vi "UDP Data Link RT Driver VI.vi"(7 "Operation":T1, 11 "Device Reference in":T2 format="%.0x") -> (0 "Error Code":i32)   [LabVIEW 2015, in "UDP Data Link Engine.lvlib"]
uses:
  UDP Data Link Engine.lvlib
  <vilib>/NI Veristand/Custom Device API/Custom Device Item Ref.ctl
  <vilib>/NI Veristand/Custom Device API/Hardware Interface Driver VI Operation.ctl
  <vilib>/NI Veristand/Custom Device API/Block Data Reference.ctl
  <vilib>/NI Veristand/Custom Device API/Data Reference.ctl
  <vilib>/NI Veristand/Custom Device API/Global Data Refs.vi
  <vilib>/NI Veristand/Custom Device API/Custom Device API.lvlib
  <vilib>/NI Veristand/Custom Device Tools/Custom Device Utility Library/Custom Device Utility Library.lvlib
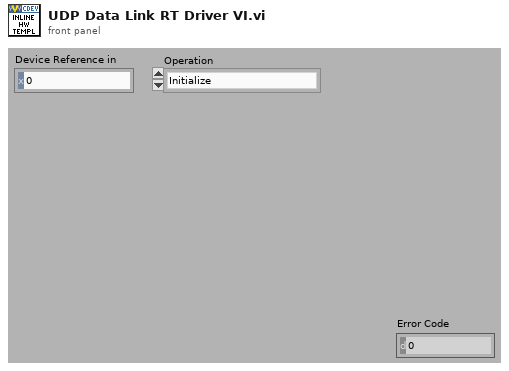
[diagram p1: front panel]
types:
  T1 = typedef "Custom Device API.lvlib/Hardware Interface Driver VI Operation.ctl" = enum16{"Initialize", "Start", "Read Data from HW", "Write Data to HW", "Close"}
  T2 = typedef "Custom Device API.lvlib/Custom Device Item Ref.ctl" = u64
  T3 = typedef "Custom Device API.lvlib/Block Data Reference.ctl" = cluster{"Data Reference":T4, "Offset":u64, "Length":u64}
  T4 = typedef "Custom Device API.lvlib/Data Reference.ctl" = i32
  T5 = cluster{"Rx FIFO Polling Rate":u32, "Rx FIFO Timeout":u32, "Tx Data Refs":cluster{"Block Data Refs":T3[], "Values Array":dbl[]}, "Rx Data Refs":cluster{"Block Data Refs":T3[], "Values Array":dbl[]}, "SeqNum FIFO Index":i32, "SeqNum Array Index":i32, "Status Notifier":refnum<notifier>, "Tx Data FIFO":refnum<k33>, "Rx Data FIFO":refnum<k33>, "error out":errorcluster, "Tx RT FIFO Timeout":bool, "Rx RT FIFO Timeout":bool}
  T6 = cluster{"read mode":enum16{"polling", "blocking"}, "write mode":enum16{"polling", "blocking"}}
  T7 = cluster{"Block Data Refs":T3[], "Values Array":dbl[]}
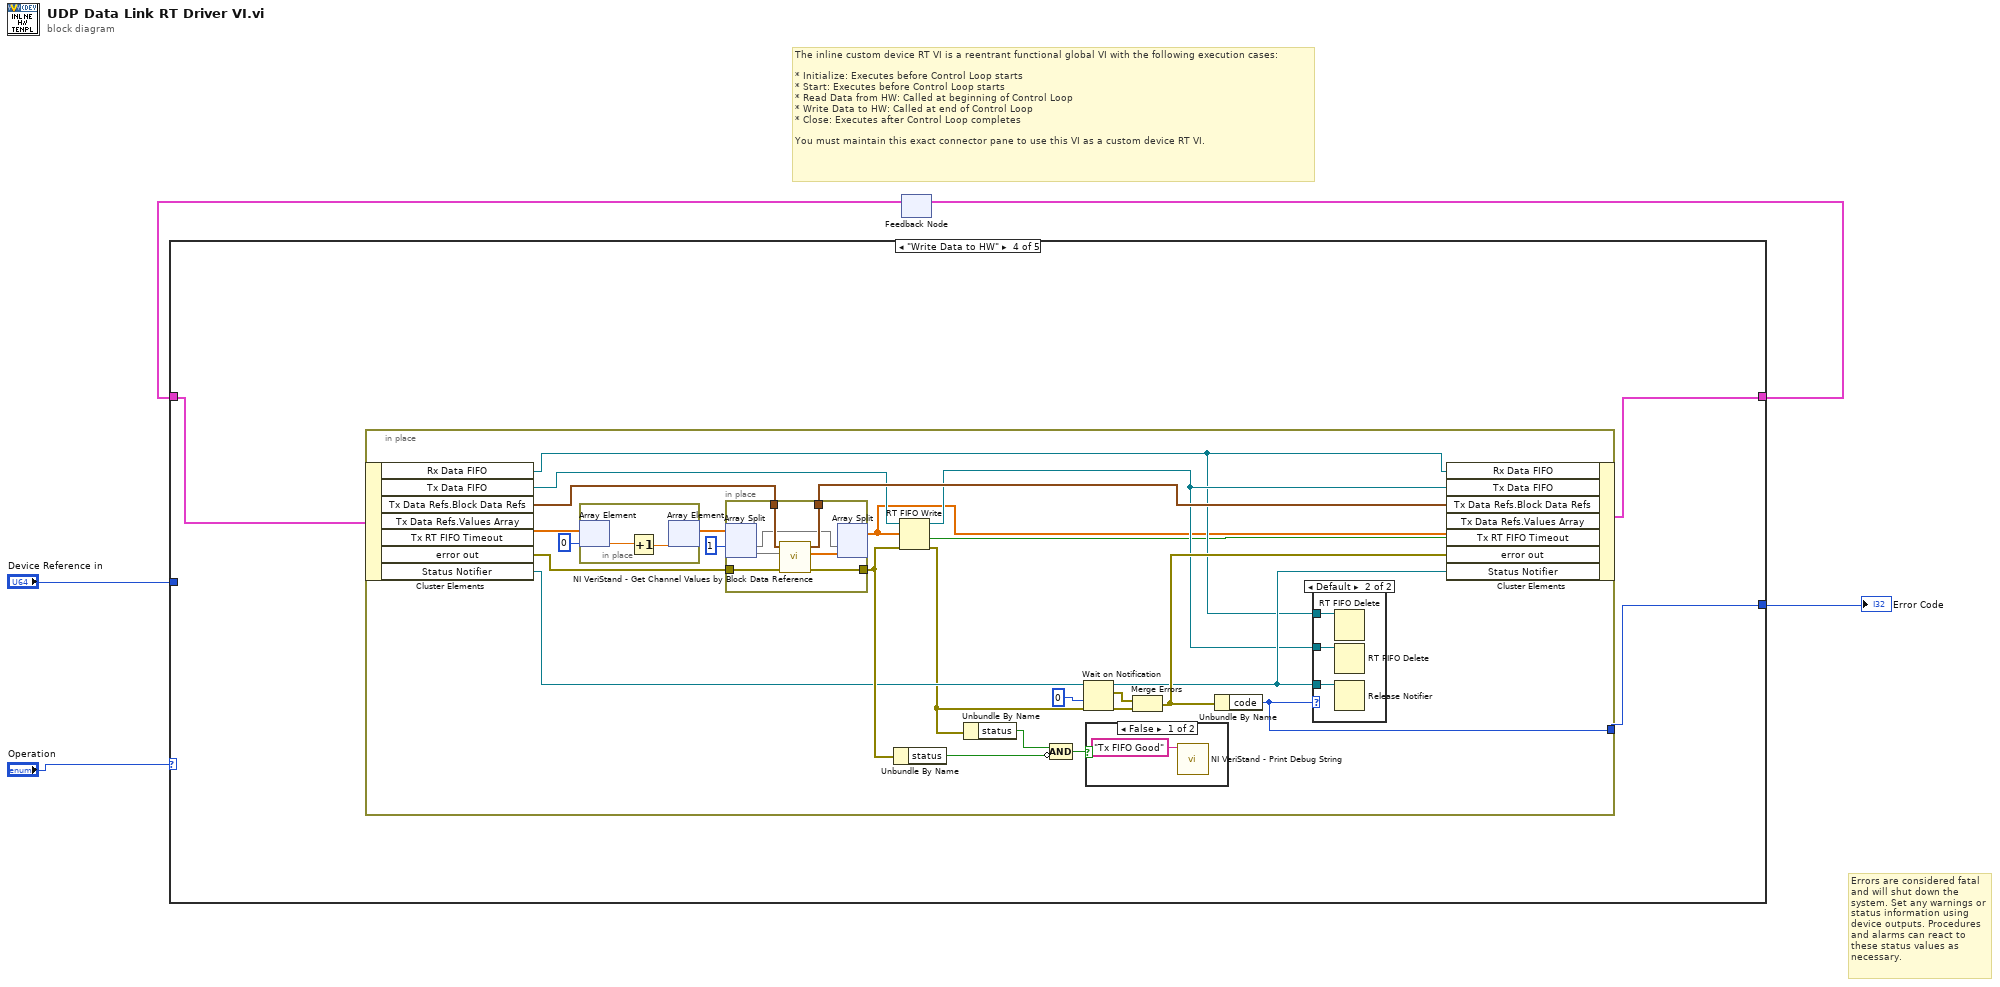
[diagram p0: block diagram]
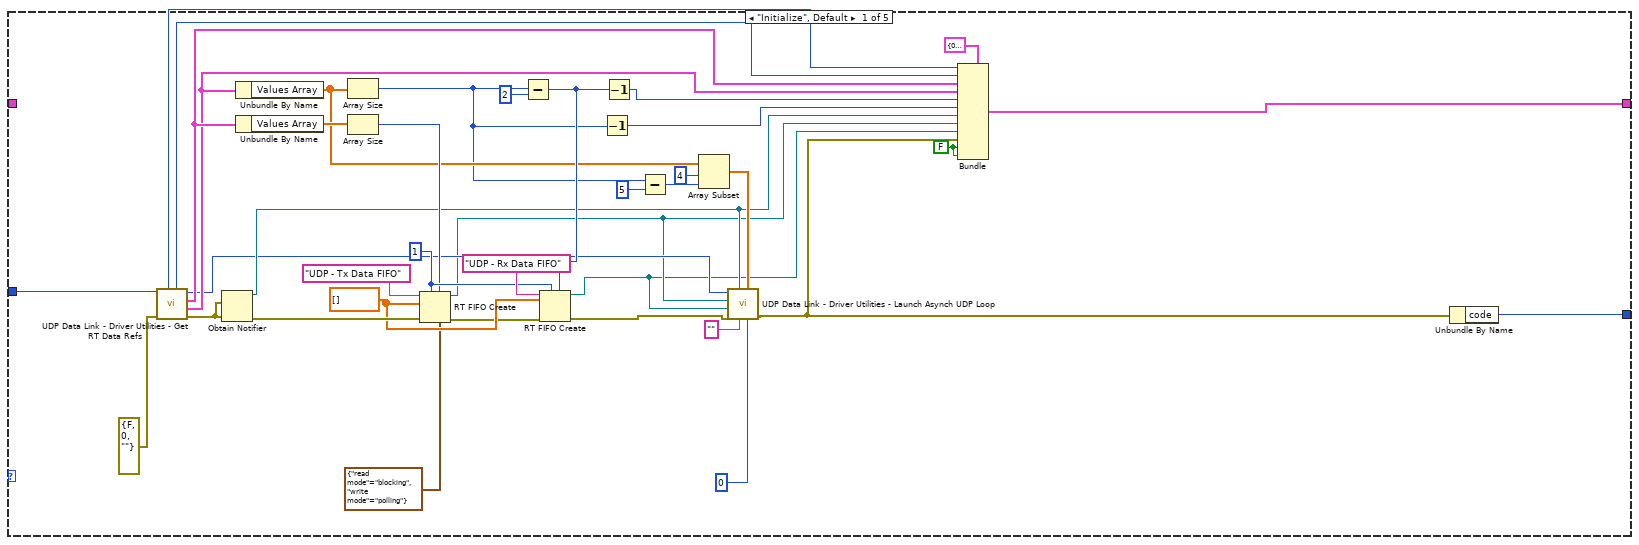
[diagram p2: hidden frame]
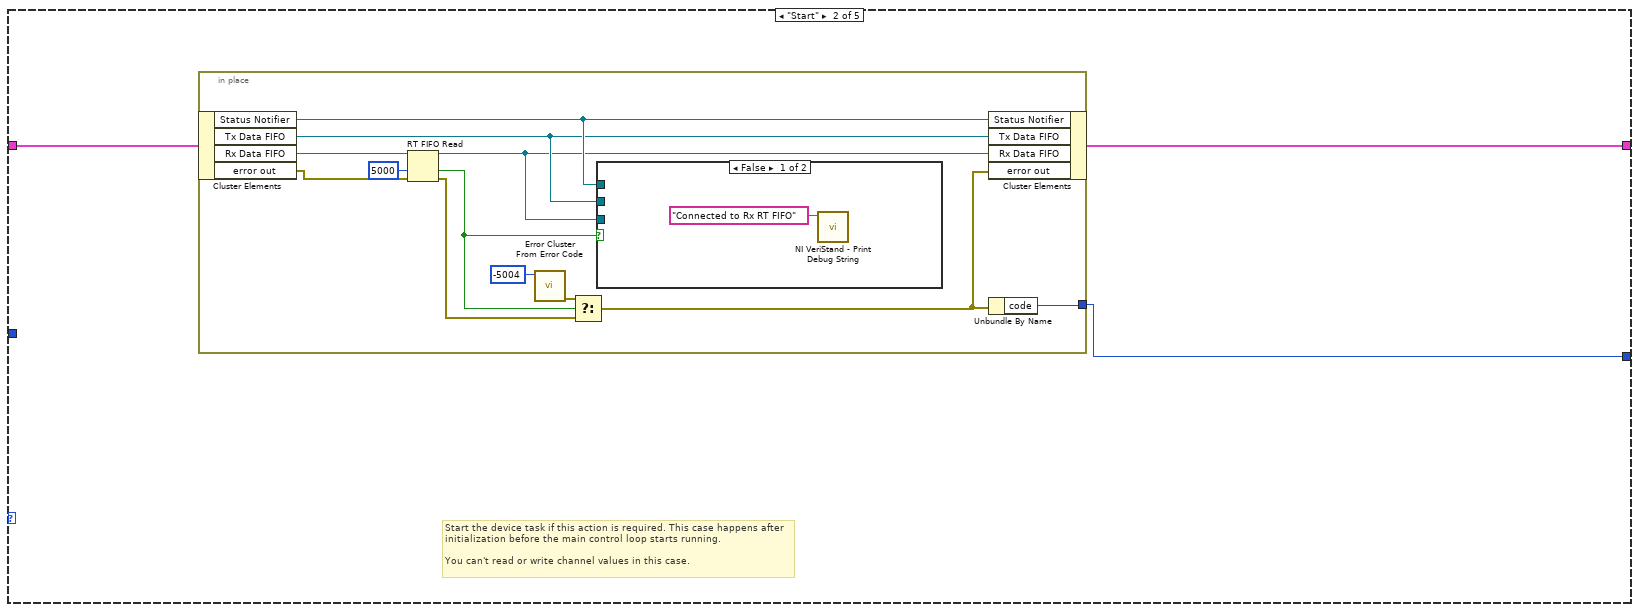
[diagram p3: hidden frame]
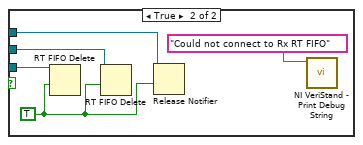
[diagram p4: hidden frame]
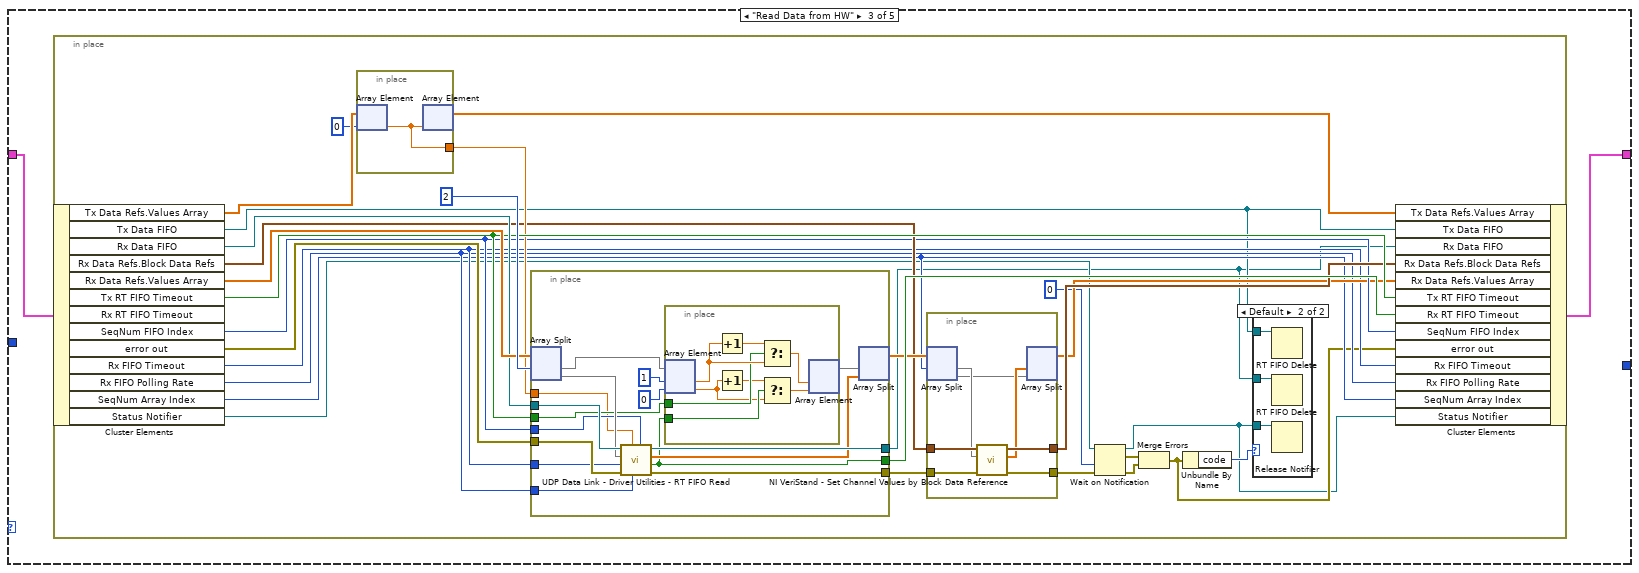
[diagram p5: hidden frame]
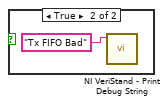
[diagram p8: hidden frame]
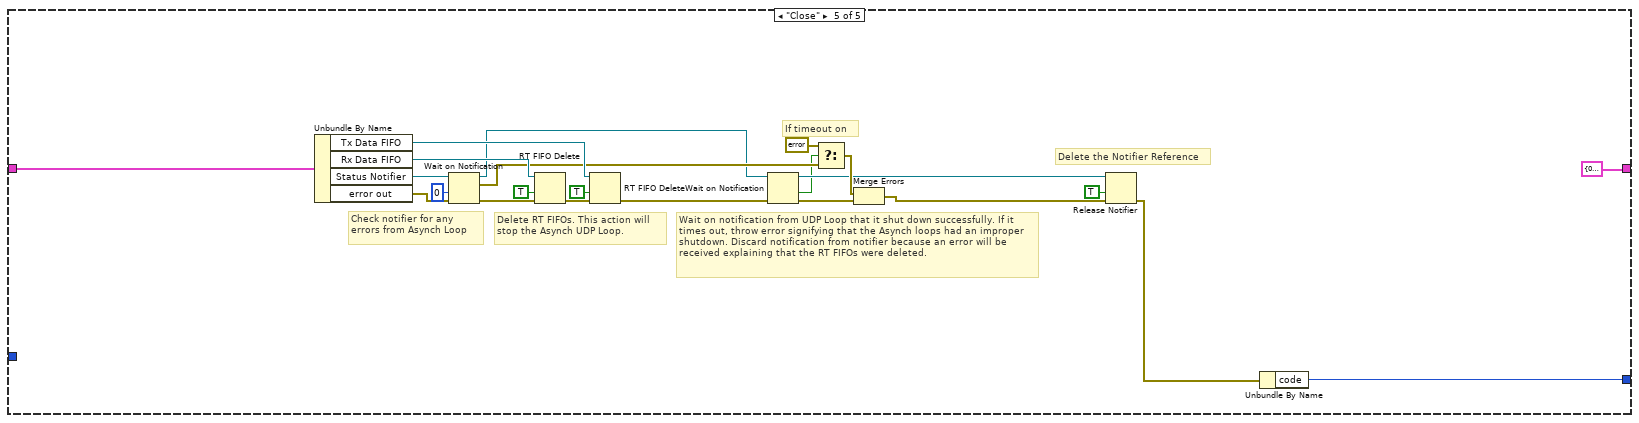
[diagram p9: hidden frame]
diagram:
  # "Errors are considered fatal and will shut down the system. Set any warnings or status information using device outputs. Procedures and alarms can react to these status values as necessary."
  # "The inline custom device RT VI is a reentrant functional global VI with the following execution cases:\n\n* Initialize: Executes before Control Loop starts\n* Start: Executes before Control Loop starts\n* Read Data from HW: Called at beginning of Control Loop\n* Write Data to HW: Called at end of Control Loop\n* Close: Executes after Control Loop completes\n\nYou must maintain this exact connector pane to use this VI as a custom device RT VI."
  n1 = feedback #1() -> (w3:T5)  [unwired: 1 out]
  n2 = case shown="\"Write Data to HW\"" "Operation" {
    tunnel: [w43 w45 w65 w131 T5 {"Rx FIFO Polling Rate"=0, "Rx FIFO Timeout"=0, "Tx Data Refs"={"Block Data Refs"=[], "Values Array"=[]}, "Rx Data Refs"={"Block Data Refs"=[], "Values Array"=[]}, "SeqNum FIFO Index"=0, "SeqNum Array Index"=0, "Status Notifier"=refnum, "Tx Data FIFO"=refnum, "Rx Data FIFO"=refnum, "error out"={"status"=FALSE, "code"=0, "source"=""}, "Tx RT FIFO Timeout"=FALSE, "Rx RT FIFO Timeout"=FALSE} ("cluster")] -> w4
    tunnel: w3 -> [_ w46 w66 w132 w175]
    tunnel: "Device Reference in" -> [w42 _ _ _ _]
    tunnel: [w29 w44 _ w133 w173] -> w1
    frame "Initialize", Default {
      w7 = FALSE ("Tx RT FIFO Timeout")
      w35 = u32 1 ("size (10)")
      w36 = dbl[] []
      n3 = call "UDP Data Link - Driver Utilities - Get RT Data Refs.vi"("error in (no error)"=errorcluster {"status"=FALSE, "code"=0, "source"=""}, "Device Ref in"=w42) -> ("error out"=w40:errorcluster, "Rx Data Refs"=w30:T7, "Tx Data Refs"=w31:T7, "Device Ref out"=w15:T2, "Rx FIFO Timeout"=w28:u32, "Rx FIFO Polling Rate"=w27:u32)  [unwired: 4 in]
      n4 = Obtain Notifier(notification data type=w40, error in (no error)=w40) -> (notifier out=w16:refnum<notifier>, error out=w39:errorcluster)  [unwired: 2 in, 1 out]
      n5 = Unbundle By Name(w30) -> ("Values Array"=w20:dbl[])
      n6 = Unbundle By Name(w31) -> ("Values Array"=w34:dbl[])
      n7 = Array Size(array=w20) -> (size(s)=w19:i32)
      n8 = Array Size(array=w34) -> (size(s)=w33:i32)
      n9 = RT FIFO Create(0:"UDP - Tx Data FIFO" ("name (unnamed)"), 1:w36, 3:w39, 4:w35, 6:w33, 7:T6 {"read mode"=enum."blocking", "write mode"=enum."polling"} ("r/w modes (polling,polling)")) -> (8:w14:refnum<k33>, 11:w9:errorcluster)  [unwired: 2 in, 1 out]
      n10 = Subtract(x=w19, y=2) -> (x-y=w26:i32)
      n11 = RT FIFO Create(0:"UDP - Rx Data FIFO" ("name (unnamed)"), 1:w36, 3:w9, 4:w35, 6:w26) -> (8:w13:refnum<k33>, 11:w8:errorcluster)  [unwired: 3 in, 1 out]
      n12 = Decrement(x=w19) -> (x-1=w25:i32)
      n13 = Decrement(x=w26) -> (x-1=w24:i32)
      n14 = Subtract(x=w19, y=5) -> (x-y=w22:i32)
      n15 = Array Subset(array=w20, index=4 ("y"), length=w22) -> (w17:dbl[])
      n16 = call "UDP Data Link - Driver Utilities - Launch Asynch UDP Loop.vi"("In4Ver"=u16 0, "Rx Initial Values"=w17, "SourceNodeName"="", "Status Notifier"=w16, "error in (no error)"=w8, "Rx Data FIFO"=w13, "Tx Data FIFO"=w14, "Device Reference in"=w15) -> ("error out"=w18:errorcluster)  [unwired: 3 in]
      n17 = Bundle(cluster=T5 {"Rx FIFO Polling Rate"=0, "Rx FIFO Timeout"=0, "Tx Data Refs"={"Block Data Refs"=[], "Values Array"=[]}, "Rx Data Refs"={"Block Data Refs"=[], "Values Array"=[]}, "SeqNum FIFO Index"=0, "SeqNum Array Index"=0, "Status Notifier"=refnum, "Tx Data FIFO"=refnum, "Rx Data FIFO"=refnum, "error out"={"status"=FALSE, "code"=0, "source"=""}, "Tx RT FIFO Timeout"=FALSE, "Rx RT FIFO Timeout"=FALSE}, "Rx FIFO Polling Rate"=w27, "Rx FIFO Timeout"=w28, "Tx Data Refs"=w31, "Rx Data Refs"=w30, "SeqNum FIFO Index"=w24, "SeqNum Array Index"=w25, "Status Notifier"=w16, "Tx Data FIFO"=w14, "Rx Data FIFO"=w13, "error out"=w18, "Tx RT FIFO Timeout"=w7, "Rx RT FIFO Timeout"=w7) -> (w43:T5)
      n18 = Unbundle By Name(w18) -> ("code"=w29:i32)
    }
    frame "Start" {
      # "Start the device task if this action is required. This case happens after initialization before the main control loop starts running.\n\nYou can't read or write channel values in this case."
      n19 = in-place {
        in-place-border: [w50] -> w44
        n20 = in-place-cluster #2(w46) -> ("Status Notifier"=w49:refnum<notifier>, "Tx Data FIFO"=w48:refnum<k33>, "Rx Data FIFO"=w57:refnum<k33>, "error out"=w58:errorcluster)
        n21 = RT FIFO Read(0:w57, 2:5000 ("timeout in ms (0)"), 3:w58) -> (8:w47:refnum<k33>, 10:w52:bool, 11:w53:errorcluster)  [unwired: 1 in, 2 out]
        n22 = call <vilib>:"Error Cluster From Error Code.vi"("error code (0)"=-5004) -> ("error out"=w54:errorcluster)  [unwired: 8 in]
        n23 = Select(t=w54, s=w52, f=w53) -> (s? t:f=w51:errorcluster)
        n24 = case shown="False" w52 {
          tunnel: w47 -> [_ w64]
          tunnel: w48 -> [_ w63]
          tunnel: w49 -> [_ w62]
          frame False {
            n25 = call <vilib>:"NI VeriStand - Print Debug String.vi"("Message"="Connected to Rx RT FIFO" ("Debug String")) -> ()  [unwired: 10 in, 1 out]
          }
          frame True {
            w61 = TRUE ("force destroy? (F)")
            n26 = RT FIFO Delete(0:w64, 2:w61) -> ()  [unwired: 1 in, 1 out]
            n27 = RT FIFO Delete(0:w63, 2:w61) -> ()  [unwired: 1 in, 1 out]
            n28 = Release Notifier(notifier=w62, force destroy? (F)=w61) -> ()  [unwired: 1 in, 3 out]
            n29 = call <vilib>:"NI VeriStand - Print Debug String.vi"("Message"="Could not connect to Rx RT FIFO" ("Debug String")) -> ()  [unwired: 10 in, 1 out]
          }
        }
        n30 = in-place-cluster #2("Status Notifier"=w49, "Tx Data FIFO"=w48, "Rx Data FIFO"=w47, "error out"=w51) -> (w45:T5)
        n31 = Unbundle By Name(w51) -> ("code"=w50:i32)
      }
    }
    frame "Read Data from HW" {
      n32 = in-place {
        n33 = in-place-cluster #3(w66) -> ("Tx Data Refs.Values Array"=w88:dbl[], "Tx Data FIFO"=w70:refnum<k33>, "Rx Data FIFO"=w93:refnum<k33>, "Rx Data Refs.Block Data Refs"=w85:T3[], "Rx Data Refs.Values Array"=w94:dbl[], "Tx RT FIFO Timeout"=w92:bool, "SeqNum FIFO Index"=w82:i32, "error out"=w90:errorcluster, "Rx FIFO Timeout"=w80:u32, "Rx FIFO Polling Rate"=w79:u32, "SeqNum Array Index"=w78:i32, "Status Notifier"=w73:refnum<notifier>)  [unwired: 1 out]
        n34 = in-place {
          in-place-border: [w99] -> w86
          n35 = in-place-array #4(w88, 0) -> (w99:dbl)
          n36 = in-place-array #4(w99) -> (w87:dbl[])  [unwired: 1 out]
        }
        n37 = in-place {
          in-place-border: w93 -> [w122]
          in-place-border: [w121] -> w69
          in-place-border: w92 -> [w115]
          in-place-border: [w114] -> w91
          in-place-border: w90 -> [w112]
          in-place-border: [w111] -> w83
          in-place-border: w80 -> [w110]
          in-place-border: w79 -> [w109]
          in-place-border: w82 -> [w108]
          in-place-border: w86 -> [w107]
          n38 = in-place-split #5(w94, 2) -> (w118:dbl[], w120:dbl[])
          n39 = call "UDP Data Link - Driver Utilities - RT FIFO Read.vi"("SeqNum FIFO Index"=w108, "poll rate in us"=w109, "Current SeqNum"=w107, "error in (no error)"=w112, "timeout in us"=w110, "element"=w120, "rt fifo (dbl array)"=w122) -> ("error out"=w111:errorcluster, "empty?"=w114:bool, "element out"=w119:dbl[], "rt fifo out (dbl array)"=w121:refnum<k33>)  [unwired: 1 out]
          n40 = in-place {
            in-place-border: w115 -> [w127]
            in-place-border: w114 -> [w126]
            n41 = in-place-array #6(w118, 1, 0) -> (w129:dbl, w124:dbl)
            n42 = Increment(x=w129) -> (x+1=w130:dbl)
            n43 = Increment(x=w124) -> (x+1=w125:dbl)
            n44 = Select(t=w130, s=w127, f=w129) -> (s? t:f=w128:dbl)
            n45 = Select(t=w125, s=w126, f=w124) -> (s? t:f=w123:dbl)
            n46 = in-place-array #6(w128, w123) -> (w113:dbl[])  [unwired: 2 out]
          }
          n47 = in-place-split #5(w113, w119) -> (w89:dbl[])  [unwired: 1 out]
        }
        n48 = in-place {
          in-place-border: w85 -> [w106]
          in-place-border: [w105] -> w84
          in-place-border: w83 -> [w101]
          in-place-border: [w100] -> w72
          n49 = in-place-split #7(w89, w78) -> (w104:dbl[], w102:dbl[])
          n50 = call <vilib>:"NI VeriStand - Set Channel Values by Block Data Reference.vi"("error in (no error)"=w101, "Values Array in"=w104, "Block Data Ref"=w106) -> ("error out"=w100:errorcluster, "Values Array out"=w103:dbl[], "Block Data Ref dup"=w105:T3[])  [unwired: 6 in]
          n51 = in-place-split #7(w103, w102) -> (w81:dbl[])  [unwired: 1 out]
        }
        n52 = Wait on Notification(notifier=w73, timeout in ms (-1)=0, error in (no error)=w72) -> (notifier out=w68:refnum<notifier>, notification=w75:errorcluster, error out=w76:errorcluster)  [unwired: 1 in, 1 out]
        n53 = Merge Errors(w75, w76) -> (w71:errorcluster)
        n54 = Unbundle By Name(w71) -> ("code"=w77:i32)
        n55 = case shown="Default" w77 {
          tunnel: w68 -> [_ w98]
          tunnel: w70 -> [_ w97]
          tunnel: w69 -> [_ w96]
          frame 0 {
          }
          frame Default {
            n56 = RT FIFO Delete(0:w97) -> ()  [unwired: 2 in, 1 out]
            n57 = RT FIFO Delete(0:w96) -> ()  [unwired: 2 in, 1 out]
            n58 = Release Notifier(notifier=w98) -> ()  [unwired: 2 in, 3 out]
          }
        }
        n59 = in-place-cluster #3("Tx Data Refs.Values Array"=w87, "Tx Data FIFO"=w70, "Rx Data FIFO"=w69, "Rx Data Refs.Block Data Refs"=w84, "Rx Data Refs.Values Array"=w81, "Tx RT FIFO Timeout"=w92, "Rx RT FIFO Timeout"=w91, "SeqNum FIFO Index"=w82, "error out"=w71, "Rx FIFO Timeout"=w80, "Rx FIFO Polling Rate"=w79, "SeqNum Array Index"=w78, "Status Notifier"=w68) -> (w65:T5)
      }
    }
    frame "Write Data to HW" {
      n60 = in-place {
        in-place-border: [w145] -> w133
        n61 = in-place-cluster #8(w132) -> ("Rx Data FIFO"=w137:refnum<k33>, "Tx Data FIFO"=w151:refnum<k33>, "Tx Data Refs.Block Data Refs"=w153:T3[], "Tx Data Refs.Values Array"=w155:dbl[], "error out"=w154:errorcluster, "Status Notifier"=w144:refnum<notifier>)  [unwired: 1 out]
        n62 = in-place {
          n63 = in-place-array #9(w155, 0) -> (w171:dbl)
          n64 = Increment(x=w171) -> (x+1=w170:dbl)
          n65 = in-place-array #9(w170) -> (w150:dbl[])  [unwired: 1 out]
        }
        n66 = in-place {
          in-place-border: [w169] -> w152
          in-place-border: [w168] -> w149
          in-place-border: w154 -> [w167]
          in-place-border: w153 -> [w166]
          n67 = in-place-split #10(w150, 1) -> (w163:dbl[], w165:dbl[])
          n68 = call <vilib>:"NI VeriStand - Get Channel Values by Block Data Reference.vi"("error in (no error)"=w167, "Values Array in"=w165, "Block Data Ref"=w166) -> ("error out"=w168:errorcluster, "Values Array out"=w164:dbl[], "Block Data Ref dup"=w169:T3[])  [unwired: 6 in]
          n69 = in-place-split #10(w163, w164) -> (w136:dbl[])  [unwired: 1 out]
        }
        n70 = Unbundle By Name(w149) -> ("status"=w146:bool)
        n71 = RT FIFO Write(0:w151, 1:w136, 3:w149) -> (8:w138:refnum<k33>, 10:w134:bool, 11:w135:errorcluster)  [unwired: 2 in, 1 out]
        n72 = Unbundle By Name(w135) -> ("status"=w147:bool)
        n73 = Compound Arithmetic op=AND(w147, invert w146) -> (w148:bool)
        n74 = Wait on Notification(notifier=w144, timeout in ms (-1)=0, error in (no error)=w135) -> (notifier out=w139:refnum<notifier>, notification=w142:errorcluster, error out=w143:errorcluster)  [unwired: 1 in, 1 out]
        n75 = case shown="False" w148 {
          frame False {
            n76 = call <vilib>:"NI VeriStand - Print Debug String.vi"("Message"="Tx FIFO Good" ("Debug String")) -> ()  [unwired: 10 in, 1 out]
          }
          frame True {
            n77 = call <vilib>:"NI VeriStand - Print Debug String.vi"("Message"="Tx FIFO Bad" ("message")) -> ()  [unwired: 10 in, 1 out]
          }
        }
        n78 = Merge Errors(w142, w143) -> (w141:errorcluster)
        n79 = Unbundle By Name(w141) -> ("code"=w145:i32)
        n80 = case shown="Default" w145 {
          tunnel: w139 -> [_ w160]
          tunnel: w138 -> [_ w159]
          tunnel: w137 -> [_ w158]
          frame 0 {
          }
          frame Default {
            n81 = RT FIFO Delete(0:w158) -> ()  [unwired: 2 in, 1 out]
            n82 = RT FIFO Delete(0:w159) -> ()  [unwired: 2 in, 1 out]
            n83 = Release Notifier(notifier=w160) -> ()  [unwired: 2 in, 3 out]
          }
        }
        n84 = in-place-cluster #8("Rx Data FIFO"=w137, "Tx Data FIFO"=w138, "Tx Data Refs.Block Data Refs"=w152, "Tx Data Refs.Values Array"=w136, "Tx RT FIFO Timeout"=w134, "error out"=w141, "Status Notifier"=w139) -> (w131:T5)
      }
    }
    frame "Close" {
      # "Delete the Notifier Reference"
      # "Wait on notification from UDP Loop that it shut down successfully. If it times out, throw error signifying that the Asynch loops had an improper shutdown. Discard notification from notifier because an error will be received explaining that the RT FIFOs were deleted."
      # "Delete RT FIFOs. This action will stop the Asynch UDP Loop."
      # "Check notifier for any errors from Asynch Loop"
      # "If timeout on"
      n85 = Unbundle By Name(w175) -> ("Tx Data FIFO"=w192:refnum<k33>, "Rx Data FIFO"=w194:refnum<k33>, "Status Notifier"=w184:refnum<notifier>, "error out"=w183:errorcluster)
      n86 = Wait on Notification(notifier=w184, timeout in ms (-1)=0, error in (no error)=w183) -> (notifier out=w179:refnum<notifier>, notification=w188:errorcluster, error out=w182:errorcluster)  [unwired: 1 in, 1 out]
      n87 = RT FIFO Delete(0:w194, 2:TRUE ("force destroy? (F)"), 3:w182) -> (11:w193:errorcluster)
      n88 = RT FIFO Delete(0:w192, 2:TRUE ("force destroy? (F)"), 3:w193) -> (11:w181:errorcluster)
      n89 = Wait on Notification(notifier=w179, error in (no error)=w181) -> (notifier out=w178:refnum<notifier>, timed out?=w177:bool, error out=w180:errorcluster)  [unwired: 2 in, 1 out]
      n90 = Select(t=errorcluster {"status"=FALSE, "code"=-5005, "source"=""}, s=w177, f=w188) -> (s? t:f=w187:errorcluster)
      n91 = Merge Errors(w187, w180) -> (w176:errorcluster)
      n92 = Release Notifier(notifier=w178, force destroy? (F)=TRUE, error in (no error)=w176) -> (error out=w174:errorcluster)  [unwired: 2 out]
      n93 = Unbundle By Name(w174) -> ("code"=w173:i32)
    }
  }
  "Error Code" <- w1
  n94 = feedback-in #1(w4) -> ()
